vi "HB_FGV.vi"(0 "HGF_FGV_Action":refnum<class "HGF_FGV_Action.lvclass">, 5 "error in (no error)":errorcluster) -> (14 "dup HGF_FGV_Action":refnum<class "HGF_FGV_Action.lvclass">, 19 "error out":errorcluster)   [LabVIEW 2009, in "HB_BaseClass_Examples.lvlib"]
doc: "This is a template for new Functional Global Variable, FGV_DB, instances.\n\nAuthor: H.Brand@gsi.de\n\nHistory:\nRevision 1.0.0.0: Jan 22, 2008 H.Brand@gsi.de; First release.\n\nCopyright 2008 GSI\n\nGesellschaft für Schwerionenforschung mbH\nPlanckstr. 1, 64291 Darmstadt, Germany\nContact: H.Brand@gsi.de or D.Beck@gsi.de\n\nThis file is part of the HGF LVOOP base class library.\n\n HGF LVOOP base class library is free software: you can redistribute it and/or modify\n it under the terms of the GNU General Public License as published by\n the Free Software Foundation, either version 3 of the License, or\n (at your option) any later version.\n\n HGF LVOOP base class library is distributed in the hope that it will be useful,\n but WITHOUT ANY WARRANTY; without even the implied warranty of\n MERCHANTABILITY or FITNESS FOR A PARTICULAR PURPOSE. See the\n GNU General Public License for more details.\n\n You should have received a copy of the GNU General Public License\n along with HGF LVOOP base class library. If not, see <http://www.gnu.org/licenses/>."
uses:
  lib.lib/HGF_LVC/HGF_BaseClasses/HGF_FGV/HGF_FGV_Action/HGF_FGV_Action.lvclass
  HB_BaseClass_Examples.lvlib
  lib.lib/HGF_LVC/HGF_BaseClasses/HGF_FGV/HGF_FGV.lvlib
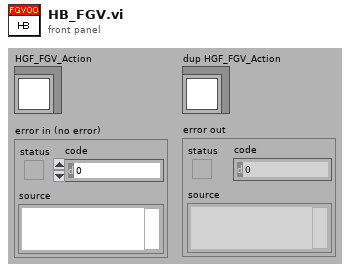
[diagram p1: front panel]
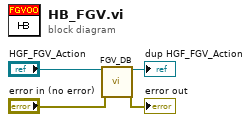
[diagram p0: block diagram]
diagram:
  n1 = call "FGV_DB.vi"("HGF_FGV_Action"="HGF_FGV_Action", "error in (no error)"="error in (no error)") -> ("dup HGF_FGV_Action"=→"dup HGF_FGV_Action":refnum<class "HGF_FGV_Action.lvclass">, "error out"=→"error out":errorcluster)  [unwired: 16 out]
